vi "Assert MemberInfo.vi"() -> ()   [LabVIEW 2015, in "Information.lvclass"]
uses:
  Information.lvclass
  API/_Database/Database.lvclass
  Information.lvclass/Information.ctl
  Member_Actor.lvlib
panel:
  in  "path":path
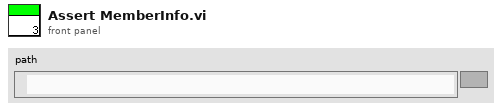
[diagram p1: front panel]
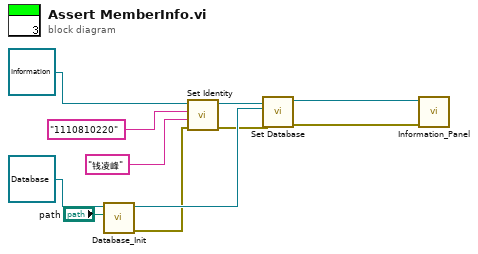
[diagram p0: block diagram]
diagram:
  n1 = call "Database_Init.vi"("path"="path", "object in"=refnum<class "Database.lvclass"> refnum ("Database")) -> ("error out"=w3:errorcluster, "object out"=w8:refnum<class "Database.lvclass">)  [unwired: 8 in]
  n2 = call "Set Identity.vi"("error in (no error)"=w3, "Name(\"\")"="钱凌峰" ("Name(\"\")"), "ID(\"\")"="1110810220" ("Name(\"\")"), "MemberInfo in"=refnum<class "Information.lvclass"> refnum) -> ("error out"=w4:errorcluster, "MemberInfo out"=w5:refnum<class "Information.lvclass">)  [unwired: 6 in]
  n3 = call "Set Database .vi"("error in (no error)"=w4, "Database"=w8, "MemberInfo in"=w5) -> ("error out"=w10:errorcluster, "MemberInfo out"=w11:refnum<class "Information.lvclass">)  [unwired: 7 in]
  n4 = call "Information_Panel.vi"("error in (no error)"=w10, "PanelController"=w11) -> ()  [unwired: 8 in, 2 out]
